vi "[GV]_Lidar 오브젝트화 제한 거리 (mm).vi"() -> ()   [LabVIEW 2016, in "Lidar Variables.lvlib"]
uses:
  Lidar Variables.lvlib
panel:
  in  "Lidar 오브젝트화 제한 거리 (mm)":dbl=200.0
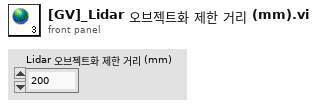
[diagram p1: front panel]
diagram:
